vi "Exponential Chirp.vi"(0 "Duration (ms)":dbl, 5 "Fmin (Hz)":dbl, 7 "Fmax (Hz)":dbl, 9 "Fs (Hz)":dbl, 11 "error in":errorcluster) -> (4 "chirp":dbl[](array[numeric]), 15 "error out":errorcluster)   [LabVIEW 2015]
uses:
  <vilib>/Analysis/1siggen.llb/Ramp Pattern by Samples.vi
  <vilib>/Analysis/3filter.llb/FIR Windowed Filter (DBL).vi
  <vilib>/Analysis/NI_AALBase.lvlib
panel:
  out "XY Graph":cluster{"Ramp Pattern":dbl[], dbl[]}(graph)
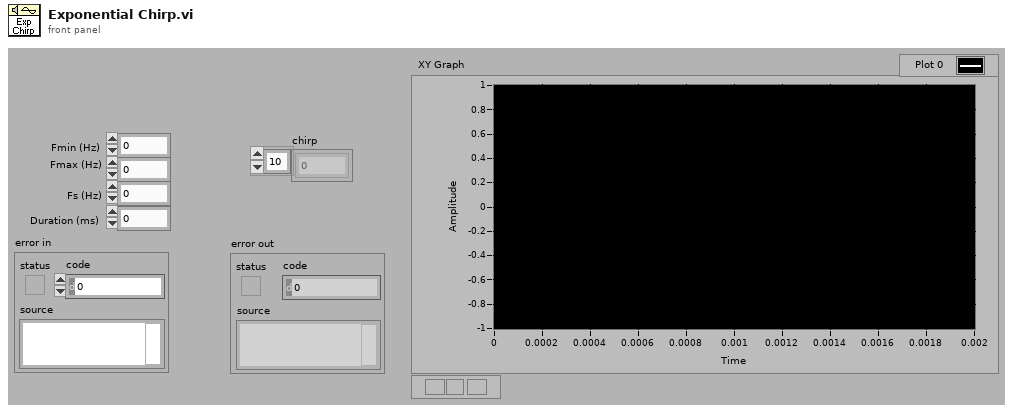
[diagram p1: front panel]
types:
  T1 = enum32{"Lowpass", "Highpass", "Bandpass", "Bandstop"}
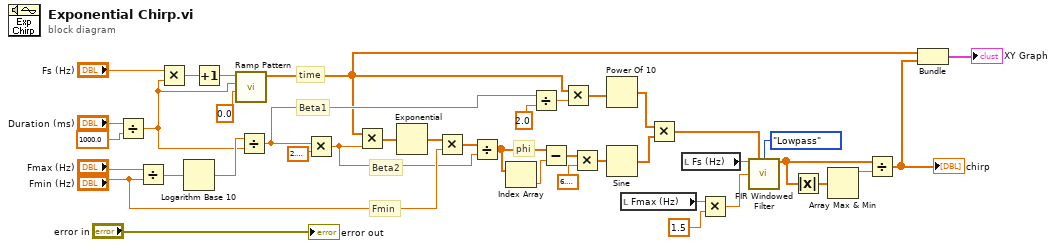
[diagram p0: block diagram]
diagram:
  # "phi"
  # "Fmin"
  # "Beta2"
  # "Beta1"
  # "time"
  n1 = Divide(x="Duration (ms)", y=1000.0 ("value")) -> (x/y=w30:dbl)
  n2 = Divide(x="Fmax (Hz)", y="Fmin (Hz)") -> (x/y=w38:dbl)
  n3 = Multiply(x="Fs (Hz)", y=w30) -> (x*y=w35:dbl)
  n4 = Logarithm Base 10(1:w38) -> (0:w31:dbl)
  n5 = Increment(x=w35) -> (x+1=w34:dbl)
  n6 = call-poly <vilib>:"Ramp Pattern.vi"("start"=0.0, "end"=w30, "samples"=w34) -> ("Ramp Pattern"=w11:dbl[])  [unwired: 7 in, 1 out]
  n7 = Divide(x=w31, y=w30) -> (x/y=w20:dbl)
  n8 = Multiply(x=w20, y=2.302585092994046) -> (x*y=w24:dbl)
  n9 = Multiply(x=w11, y=w24) -> (x*y=w28:dbl[])
  n10 = Exponential(1:w28) -> (0:w27:dbl[])
  n11 = Multiply(x=w27, y="Fmin (Hz)") -> (x*y=w25:dbl[])
  n12 = Divide(x=w25, y=w24) -> (x/y=w23:dbl[])
  n13 = Index Array(array=w23) -> (element=w22:dbl)  [unwired: 1 in]
  n14 = Divide(x=w20, y=2.0) -> (x/y=w18:dbl)
  n15 = Subtract(x=w23, y=w22) -> (x-y=w15:dbl[])
  n16 = Multiply(x=w11, y=w18) -> (x*y=w17:dbl[])
  n17 = Multiply(x=w15, y=6.283185307179586) -> (x*y=w21:dbl[])
  n18 = Power Of 10(x=w17) -> (10^x=w12:dbl[])
  n19 = Sine(x=w21) -> (sin(x)=w13:dbl[])
  n20 = local read "Fmax (Hz)"() -> (w7:dbl)
  n21 = Multiply(x=w12, y=w13) -> (x*y=w10:dbl[])
  n22 = local read "Fs (Hz)"() -> (w8:dbl)
  n23 = Multiply(x=w7, y=1.5) -> (x*y=w5:dbl)
  n24 = call-poly <vilib>:"FIR Windowed Filter.vi"("sampling freq: fs"=w8, "X"=w10, "filter type"=T1."Lowpass", "low cutoff freq: fl"=w5) -> ("Filtered X"=w4:dbl[])  [unwired: 10 in, 1 out]
  n25 = Absolute Value(x=w4) -> (abs(x)=w2:dbl[])
  n26 = Array Max & Min(array=w2) -> (max value=w3:dbl)  [unwired: 3 out]
  n27 = Divide(x=w4, y=w3) -> (x/y=w1:dbl[])
  "chirp" <- w1
  n28 = Bundle("Ramp Pattern"=w11, w1) -> (→"XY Graph":cluster{"Ramp Pattern":dbl[], dbl[]})  [unwired: 1 in]
  "error out" <- "error in"
